vi "TwGetPeakDataLV.vi"(0 "error in (no error)":errorcluster, 1 "filename":string, 6 "peakOffset":i32, 7 "peakCount":i32, 8 "segOffset":i32, 9 "segCount":i32, 10 "bufOffset":i32, 11 "bufCount":i32, 12 "writeOffset":i32, 13 "writeCount":i32) -> (14 "error out":errorcluster, 19 "dataBuffer":sgl[](array[numeric]))   [LabVIEW 2009]
uses:
  TwH5Dll.dll
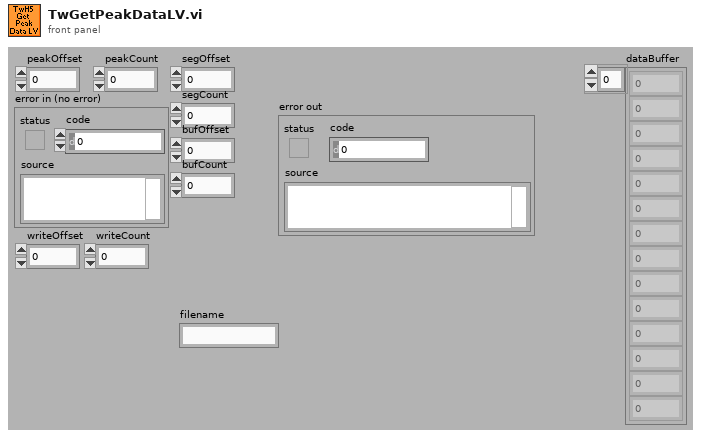
[diagram p1: front panel]
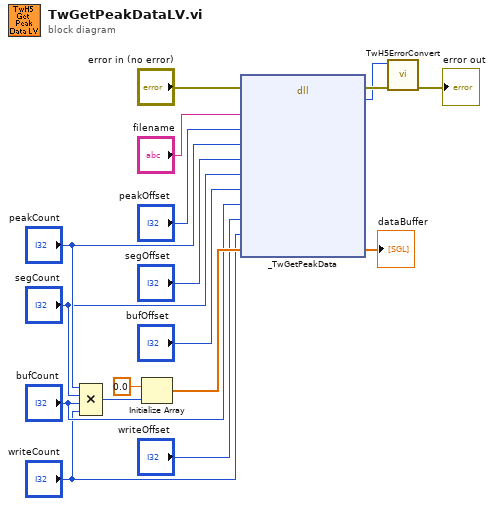
[diagram p0: block diagram]
diagram:
  n1 = Compound Arithmetic op=MULTIPLY("peakCount", "segCount", "bufCount", "writeCount") -> (w1:i32)
  n2 = Initialize Array(sgl 0.0 ("element"), w1) -> (w7:sgl[])
  n3 = dll-call lib="C:/src/85_TofDaq_current/DllWrappers/LabView/TwH5Dll/TwH5Dll.dll" fn="_TwGetPeakData"(error in="error in (no error)", "filename"="filename", "peakOffset"="peakOffset", "peakCount"="peakCount", "segOffset"="segOffset", "segCount"="segCount", "bufOffset"="bufOffset", "bufCount"="bufCount", "writeOffset"="writeOffset", "writeCount"="writeCount", "dataBuffer"=w7) -> (error out=w16:errorcluster, "TwRetVal"=w15:i32, "dataBuffer"=→"dataBuffer":sgl[])  [unwired: 11 in, 1 out]
  n4 = call "TwH5ErrorConvert.vi"("error in (no error)"=w16, "error code"=w15) -> ("error out"=→"error out":errorcluster)  [unwired: 9 out]
